vi "adjust_session_paths.vi"(2 "Sample_Information In":T2, 4 "top_level":path) -> (0 "MostRecentSessionOut":T1, 1 "Sample_Information_out":T2)   [LabVIEW 2011]
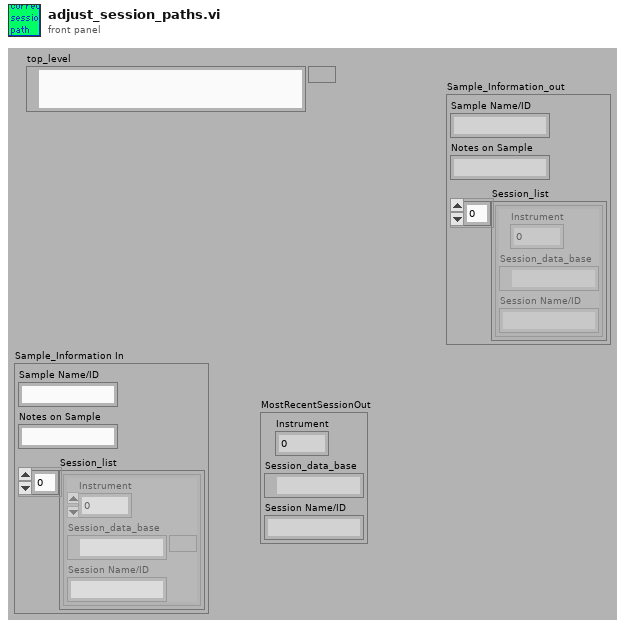
[diagram p1: front panel]
types:
  T1 = cluster{"Instrument":u16, "Session_data_base":path, "Session Name/ID":string}
  T2 = cluster{"Sample Name/ID":string, "Notes on Sample":string, "Session_list":cluster{"Instrument":u16, "Session_data_base":path, "Session Name/ID":string}[]}
  T3 = cluster{"Instrument":u16, "Session_data_base":path, "Session Name/ID":string}[]
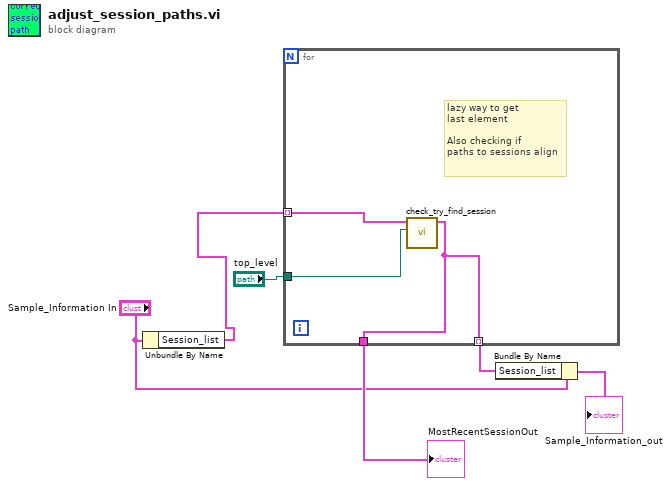
[diagram p0: block diagram]
diagram:
  n1 = Unbundle By Name("Sample_Information In") -> ("Session_list"=w1:T3)
  n2 = for {
    tunnel: w1 -> [w8] mode=indexing
    tunnel: [w7] -> w3
    tunnel: "top_level" -> [w9]
    tunnel: [w7] -> w5 mode=indexing
    # "lazy way to get\nlast element\n\nAlso checking if \npaths to sessions align"
    n3 = call "check_try_find_session.vi"("main_db_path"=w9, "Sesions"=w8) -> ("SessionOut"=w7:T1)  [unwired: 5 in]
  }
  "MostRecentSessionOut" <- w3
  n4 = Bundle By Name(cluster="Sample_Information In", "Session_list"=w5) -> (→"Sample_Information_out":T2)
